vi "MatLabVariableNames.vi"() -> (2 "systemVariableNames":string[](array[string]), 3 "userInputVariableNames":string[](array[string]))   [LabVIEW 2020]
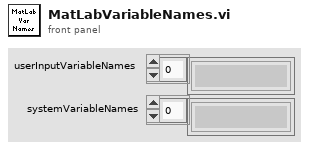
[diagram p1: front panel]
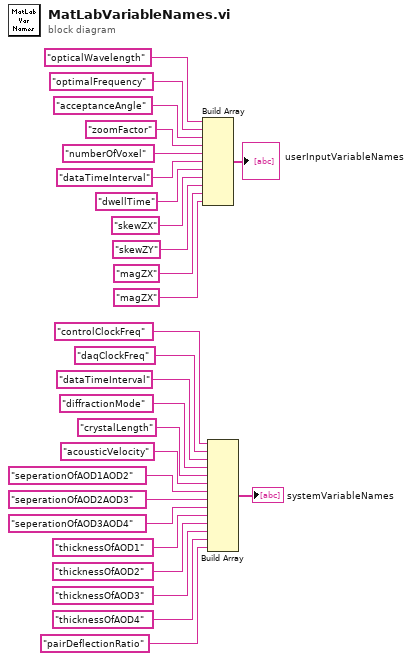
[diagram p0: block diagram]
diagram:
  n1 = Build Array("opticalWavelength", "optimalFrequency", "acceptanceAngle", "zoomFactor", "numberOfVoxel", "dataTimeInterval", "dwellTime", "skewZX", "skewZY", "magZX", "magZX") -> (→"userInputVariableNames":string[])
  n2 = Build Array("controlClockFreq", "daqClockFreq", "dataTimeInterval", "diffractionMode", "crystalLength", "acousticVelocity", "seperationOfAOD1AOD2", "seperationOfAOD2AOD3", "seperationOfAOD3AOD4", "thicknessOfAOD1", "thicknessOfAOD2", "thicknessOfAOD3", "thicknessOfAOD4", "pairDeflectionRatio") -> (→"systemVariableNames":string[])
